vi "Test Pause.vi"(11 "Error in":errorcluster) -> (15 "Error out":errorcluster)   [LabVIEW 2020, in "StopWatchTests.lvlib"]
doc: "This VI is used for validating pause button in stopwatch"
uses:
  StopWatchTests.lvlib
  <vilib>/SLL Drona/APIs/Stimulus/ControlValue/SetValueAuto.vi
  <vilib>/SLL Drona/APIs/Get/GetControlValue/GetControlValueByPathString.vi
  <vilib>/SLL Drona/APIs/Assert/AssertControlValue/Equal.vi
  <vilib>/SLL Drona/APIs/Stimulus/VI/CloseVI.vi
  <vilib>/addons/_JKI Toolkits/Caraya/classes/Test/Test.lvclass
  <vilib>/SLL Drona/Drona.lvlib
  <vilib>/SLL Drona/APIs/Stimulus/ControlValue/ControlValue.lvlib
  <vilib>/SLL Drona/APIs/Get/GetControlValue/GetControlValue.lvlib
  <vilib>/SLL Drona/APIs/Assert/AssertControlValue/AssertControlValue.lvlib
  <vilib>/SLL Drona/APIs/Stimulus/VI/VI.lvlib
panel:
  # "PAUSE TEST"
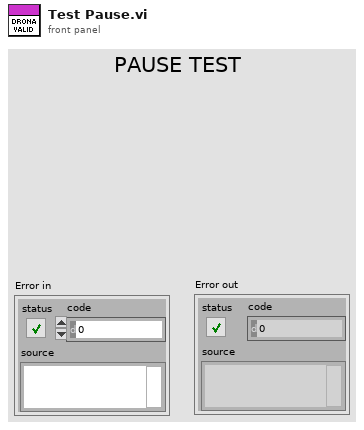
[diagram p1: front panel]
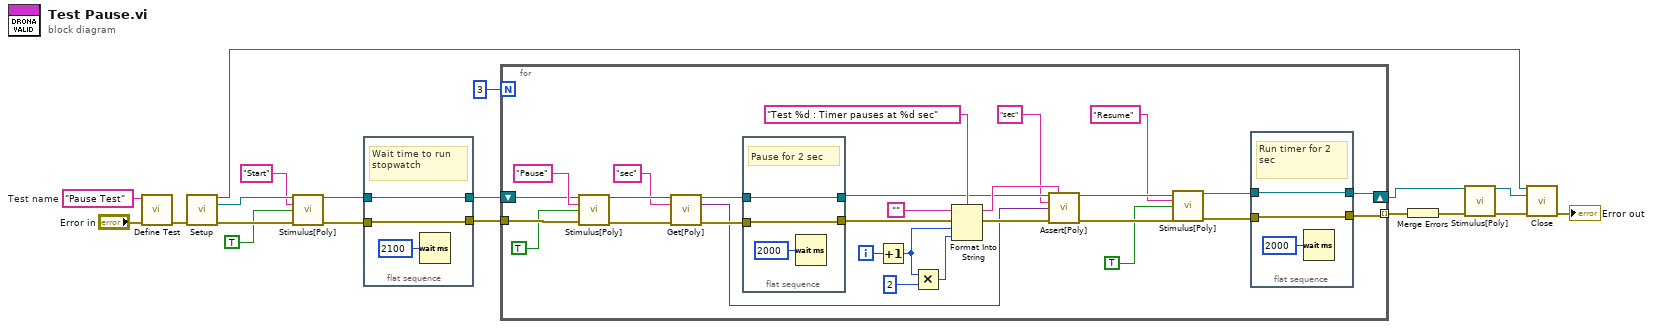
[diagram p0: block diagram]
diagram:
  w18 = "Pause Test"  # Test name
  n1 = call <vilib>:"Define Test.vi"("error in (no error)"="Error in", "Label (VI Title)"=w18) -> ("error out"=w17:errorcluster)  [unwired: 9 in]
  n2 = call <vilib>:"Setup.vi"("error in"=w17) -> ("Application Ref"=w15:refnum<vi>, "VI Reference Out"=w10:refnum<vi>, "error out"=w11:errorcluster)  [unwired: 12 in]
  n3 = call-poly <vilib>:"Stimulus[Poly].vi"("VI Reference In"=w10, "Control Path"="Start", "Value (Signaling)"=TRUE, "error in"=w11) -> ("VI Reference Out"=w6:refnum<vi>, "error out"=w7:errorcluster)  [unwired: 10 in]
  n4 = flat-sequence {
    tunnel: w7 -> [w21]
    tunnel: [w21] -> w5
    tunnel: w6 -> [w20]
    tunnel: [w20] -> w1
    frame #0 {
      # "Wait time to run  stopwatch"
      n5 = Wait (ms)(milliseconds to wait=u32 2100) -> ()  [unwired: 1 out]
    }
  }
  n6 = for {
    N: 3 -> [_]
    tunnel: w5 -> [w51]
    shift-right: [w31] -> w2
    shift-left: w1 -> [w29]
    tunnel: [w30] -> w4 mode=indexing
    i -> [w44]
    n7 = call-poly <vilib>:"Stimulus[Poly].vi"("VI Reference In"=w29, "Control Path"="Pause", "Value (Signaling)"=TRUE, "error in"=w51) -> ("VI Reference Out"=w25:refnum<vi>, "error out"=w28:errorcluster)  [unwired: 10 in]
    n8 = call-poly <vilib>:"Get[Poly].vi"("VI Reference In"=w25, "Control Path"="sec", "error in"=w28) -> ("VI Reference Out"=w26:refnum<vi>, "Value"=w23:variant, "error out"=w27:errorcluster)  [unwired: 10 in]
    n9 = flat-sequence {
      tunnel: w27 -> [w56]
      tunnel: [w56] -> w48
      tunnel: w26 -> [w55]
      tunnel: [w55] -> w42
      frame #0 {
        # "Pause for 2 sec"
        n10 = Wait (ms)(milliseconds to wait=u32 2000) -> ()  [unwired: 1 out]
      }
    }
    n11 = Increment(x=w44) -> (x+1=w40:i32)
    n12 = Multiply(x=w40, y=2) -> (x*y=w38:i32)
    n13 = Format Into String(format string="Test %d : Timer pauses at %d sec", initial string="", error in=w48, w40, w38) -> (resulting string=w43:string, error out=w47:errorcluster)
    n14 = call-poly <vilib>:"Assert[Poly].vi"("VI Reference In"=w42, "Test Label"=w43, "Control Path"="sec", "Control Value"=w23, "Error In"=w47) -> ("VI Reference Out"=w37:refnum<vi>, "Error Out"=w36:errorcluster)  [unwired: 9 in]
    n15 = call-poly <vilib>:"Stimulus[Poly].vi"("VI Reference In"=w37, "Control Path"="Resume", "Value (Signaling)"=TRUE, "error in"=w36) -> ("VI Reference Out"=w32:refnum<vi>, "error out"=w33:errorcluster)  [unwired: 10 in]
    n16 = flat-sequence {
      tunnel: w33 -> [w53]
      tunnel: [w53] -> w30
      tunnel: w32 -> [w52]
      tunnel: [w52] -> w31
      frame #0 {
        # "Run timer for 2 sec"
        n17 = Wait (ms)(milliseconds to wait=u32 2000) -> ()  [unwired: 1 out]
      }
    }
  }
  n18 = Merge Errors(w4) -> (w3:errorcluster)
  n19 = call-poly <vilib>:"Stimulus[Poly].vi"("VI Reference In"=w2, "error in"=w3) -> ("VI Reference Out"=w14:refnum<vi>, "error out"=w13:errorcluster)  [unwired: 12 in]
  n20 = call <vilib>:"Close.vi"("Application Ref"=w15, "VI Reference"=w14, "error in"=w13) -> ("error out"=→"Error out":errorcluster)  [unwired: 12 in]
